vi "Result.vi"(0 "SystemEvents in":refnum<class "SystemEvents.lvclass">, 1 "event data":T1, 5 "error in (no error)":errorcluster) -> (14 "SystemEvents out":refnum<class "SystemEvents.lvclass">, 19 "error out":errorcluster)   [LabVIEW 2017, in "SystemEvents.lvclass"]
doc: "Fires the Result event with the input parameters in attributes of the event data variant."
uses:
  SystemEvents.lvclass
  SystemEventData/ResultEventData.ctl
  SystemEventData/ResultType.ctl
  SystemEvents.lvclass/SystemEvents.ctl
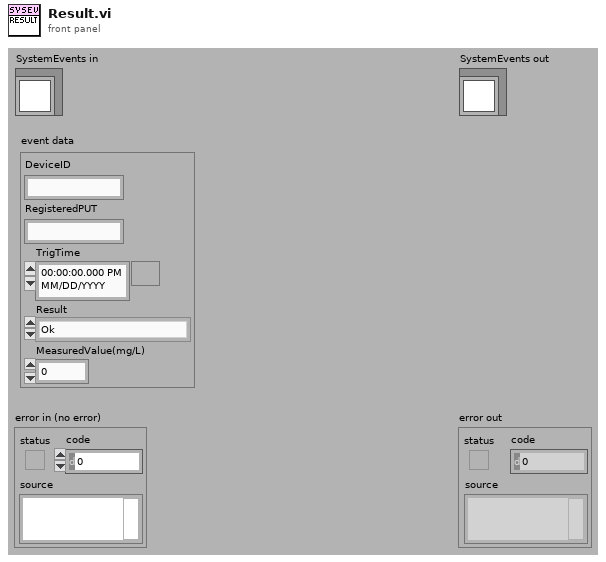
[diagram p1: front panel]
types:
  T1 = typedef "ResultEventData.ctl" = cluster{"DeviceID":string, "RegisteredPUT":string, "TrigTime":timestamp, "Result":T2, "MeasuredValue(mg/L)":dbl}
  T2 = typedef "ResultType.ctl" = enum16{"Ok", "Outside limits", "Bad reading", "CtrlMeas OK", "CtrlMeas Not OK"}
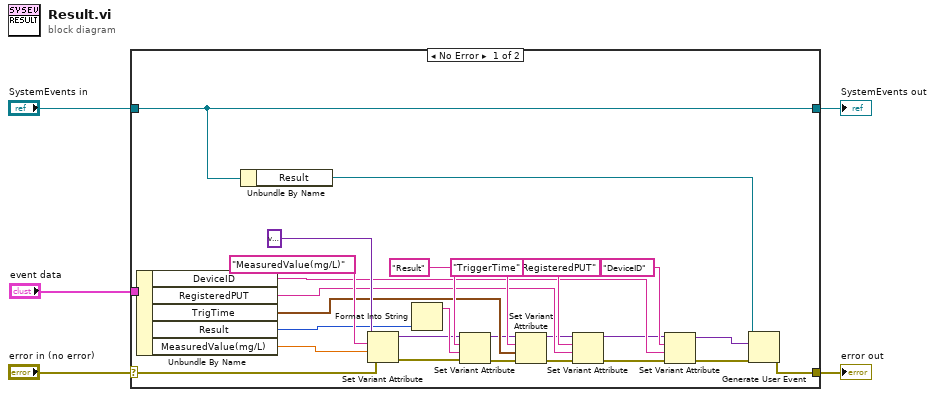
[diagram p0: block diagram]
diagram:
  n1 = case shown="No Error" "error in (no error)" {
    selector: "error in (no error)" -> [w7 w34]
    tunnel: [w31 w34] -> w4
    tunnel: [w32 w33] -> w2
    tunnel: "SystemEvents in" -> [w32 w33]
    tunnel: "event data" -> [w28 _]
    frame No Error {
      n2 = Unbundle By Name(w28) -> ("DeviceID"=w14:string, "RegisteredPUT"=w17:string, "TrigTime"=w21:timestamp, "Result"=w25:T2, "MeasuredValue(mg/L)"=w26:dbl)
      n3 = Unbundle By Name(w32) -> ("Result"=w30:refnum<user-event>)
      n4 = Set Variant Attribute(Variant=variant, name="MeasuredValue(mg/L)", value=w26, error in=w7) -> (Variant out=w22:variant, error out=w12:errorcluster)  [unwired: 1 out]
      n5 = Format Into String(w25) -> (resulting string=w24:string)  [unwired: 3 in, 1 out]
      n6 = Set Variant Attribute(Variant=w22, name="Result", value=w24, error in=w12) -> (Variant out=w19:variant, error out=w11:errorcluster)  [unwired: 1 out]
      n7 = Set Variant Attribute(Variant=w19, name="TriggerTime", value=w21, error in=w11) -> (Variant out=w16:variant, error out=w10:errorcluster)  [unwired: 1 out]
      n8 = Set Variant Attribute(Variant=w16, name="RegisteredPUT", value=w17, error in=w10) -> (Variant out=w13:variant, error out=w9:errorcluster)  [unwired: 1 out]
      n9 = Set Variant Attribute(Variant=w13, name="DeviceID", value=w14, error in=w9) -> (Variant out=w8:variant, error out=w6:errorcluster)  [unwired: 1 out]
      n10 = Generate User Event(user event=w30, event data cluster=w8, error in=w6) -> (error out=w31:errorcluster)  [unwired: 1 in, 1 out]
    }
    frame Error {
    }
  }
  "error out" <- w4
  "SystemEvents out" <- w2
